vi "LMS_Open.vi"(8 "error in (no error)":errorcluster, 10 "lms_info_str_t":string) -> (0 "error out":errorcluster, 3 "device":i64)   [LabVIEW 2018, in "LMS_LV_Drv.lvlib"]
uses:
  LMS_LV_Drv.lvlib
  C:/Program Files/PothosSDR/bin/LimeSuite.dll
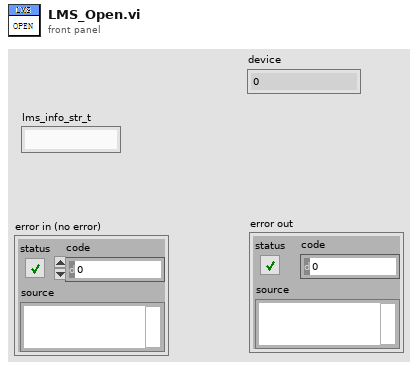
[diagram p1: front panel]
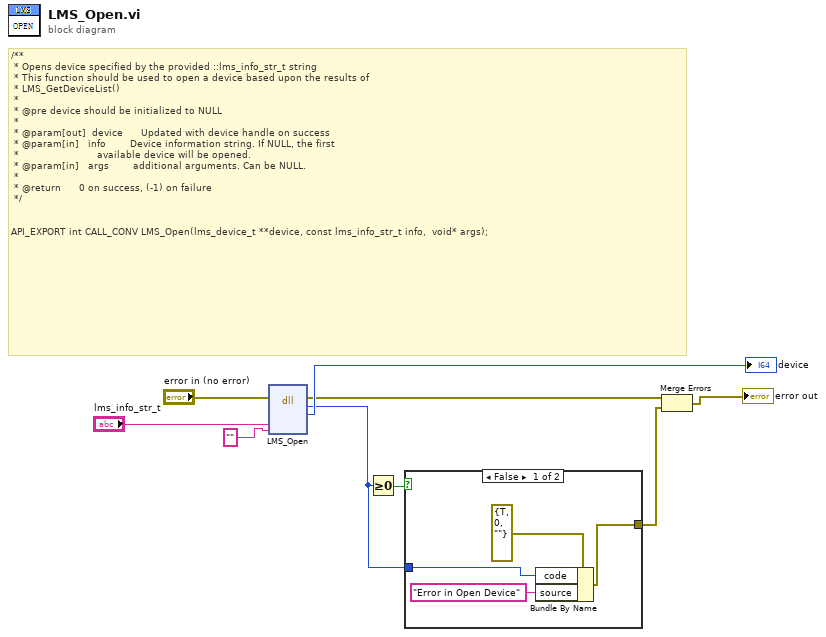
[diagram p0: block diagram]
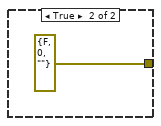
[diagram p2: hidden frame]
diagram:
  # "/**\n * Opens device specified by the provided ::lms_info_str_t string\n * This function should be used to open a device based upon the results of\n * LMS_GetDeviceList()\n *\n * @pre device should be initialized to NULL\n *\n * @param[out]  device      Updated with device handle on success\n * @param[in]   info        Device information string. If NULL, the first\n *                          available device will be opened.\n * @param[in]   args        additional arguments. Can be NULL.\n *\n * @return      0 on success, (-1) on failure\n */\n\n\nAPI_EXPORT int CALL_CONV LMS_Open(lms_device_t **device, const lms_info_str_t info,  void* args);"
  n1 = dll-call lib="C:/Program Files/PothosSDR/bin/LimeSuite.dll" fn="LMS_Open"(error in="error in (no error)", "lms_info_str_t"="lms_info_str_t", "args"="" ("lms_info_str_t")) -> (error out=w5:errorcluster, "return type"=w1:i32, "device"=→"device":i64)  [unwired: 5 in, 1 out]
  n2 = Greater Or Equal To 0?(x=w1) -> (x >= 0?=w3:bool)
  n3 = case shown="False" w3 {
    tunnel: [w12 errorcluster {"status"=FALSE, "code"=0, "source"=""} ("error in")] -> w2
    tunnel: w1 -> [w11 _]
    frame False {
      n4 = Bundle By Name(cluster=errorcluster {"status"=TRUE, "code"=0, "source"=""} ("error in"), "code"=w11, "source"="Error in Open Device") -> (w12:errorcluster)
    }
    frame True {
    }
  }
  n5 = Merge Errors(w5, w2) -> (→"error out":errorcluster)
